vi "deleave.vi"(11 "Data":u64[](array[numeric])) -> (2 "Counts":i16[][](array[numeric]), 3 "Voltage":dbl[][](array[numeric]))   [LabVIEW 2015]
doc: "Deleave and convert Data. Deleaves data from DMA readout and converts with SubVIs to counts and voltages."
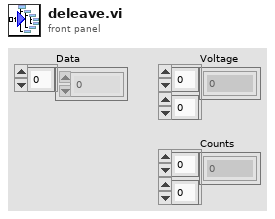
[diagram p1: front panel]
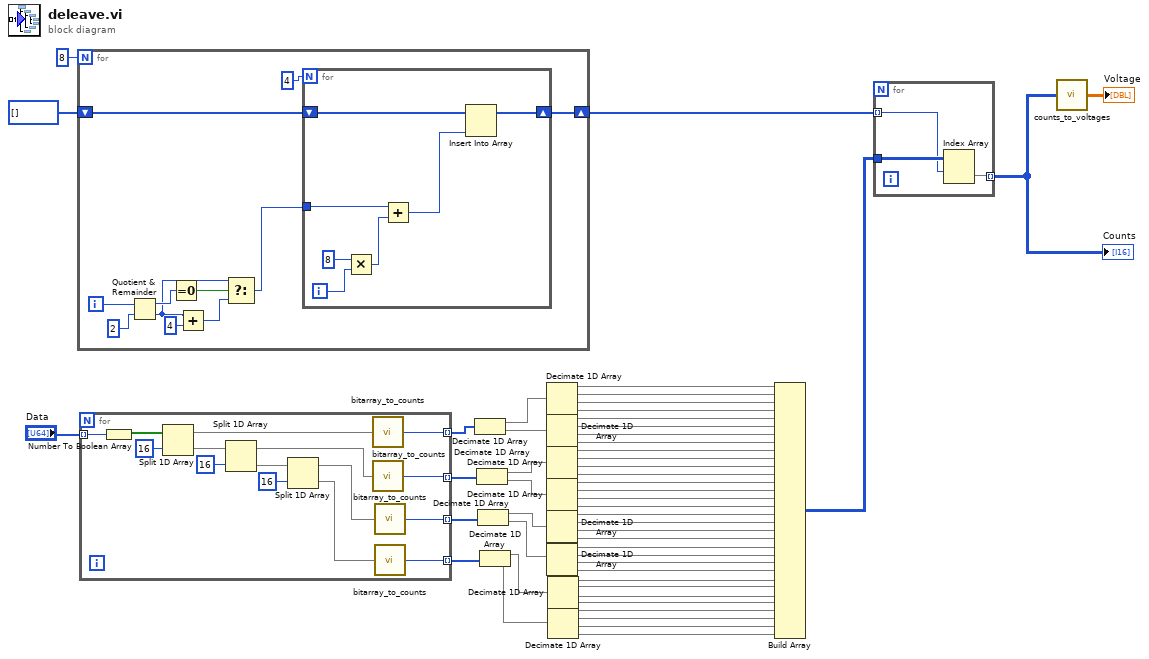
[diagram p0: block diagram]
diagram:
  n1 = for {
    N: 8 -> [_]
    shift-right: [w60] -> w2
    shift-left: i32[] [] -> [w61]
    i -> [w59]
    n2 = Quotient & Remainder(x=w59, y=2) -> (x-y*floor(x/y)=w57:i32, floor(x/y)=w52:i32)
    n3 = Equal To 0?(x=w57) -> (x = 0?=w55:bool)
    n4 = Add(x=w52, y=4) -> (x+y=w54:i32)
    n5 = Select(t=w52, s=w55, f=w54) -> (s? t:f=w53:i32)
    n6 = for {
      N: 4 -> [_]
      shift-right: [w64] -> w60
      shift-left: w61 -> [w65]
      tunnel: w53 -> [w69]
      i -> [w68]
      n7 = Multiply(x=8, y=w68) -> (x*y=w66:i32)
      n8 = Add(x=w69, y=w66) -> (x+y=w63:i32)
      n9 = Insert Into Array(array=w65, new element=w63) -> (w64:i32[])  [unwired: 1 in]
    }
  }
  n10 = for {
    tunnel: "Data" -> [w84] mode=indexing
    tunnel: [w76] -> w7 mode=indexing
    tunnel: [w74] -> w8 mode=indexing
    tunnel: [w72] -> w9 mode=indexing
    tunnel: [w71] -> w10 mode=indexing
    n11 = Number To Boolean Array(number=w84) -> (Boolean array=w83:bool[])
    n12 = Split 1D Array(array=w83, index=16) -> (first subarray=w77:bool[], second subarray=w81:bool[])
    n13 = Split 1D Array(array=w81, index=16) -> (first subarray=w75:bool[], second subarray=w78:bool[])
    n14 = Split 1D Array(array=w78, index=16) -> (first subarray=w73:bool[], second subarray=w70:bool[])
    n15 = call "bitarray_to_counts.vi"("16Bit Array"=w77) -> ("Counts"=w76:i16)
    n16 = call "bitarray_to_counts.vi"("16Bit Array"=w75) -> ("Counts"=w74:i16)
    n17 = call "bitarray_to_counts.vi"("16Bit Array"=w73) -> ("Counts"=w72:i16)
    n18 = call "bitarray_to_counts.vi"("16Bit Array"=w70) -> ("Counts"=w71:i16)
  }
  n19 = Decimate 1D Array(w7) -> (w11:i16[], w12:i16[])
  n20 = Decimate 1D Array(w8) -> (w14:i16[], w13:i16[])
  n21 = Decimate 1D Array(w9) -> (w15:i16[], w16:i16[])
  n22 = Decimate 1D Array(w10) -> (w17:i16[], w18:i16[])
  n23 = Decimate 1D Array(w11) -> (w19:i16[], w20:i16[], w21:i16[], w22:i16[])
  n24 = Decimate 1D Array(w12) -> (w23:i16[], w24:i16[], w25:i16[], w26:i16[])
  n25 = Decimate 1D Array(w14) -> (w27:i16[], w28:i16[], w29:i16[], w30:i16[])
  n26 = Decimate 1D Array(w13) -> (w31:i16[], w32:i16[], w33:i16[], w34:i16[])
  n27 = Decimate 1D Array(w15) -> (w35:i16[], w36:i16[], w37:i16[], w38:i16[])
  n28 = Decimate 1D Array(w16) -> (w39:i16[], w40:i16[], w41:i16[], w42:i16[])
  n29 = Decimate 1D Array(w17) -> (w43:i16[], w44:i16[], w45:i16[], w46:i16[])
  n30 = Decimate 1D Array(w18) -> (w47:i16[], w48:i16[], w49:i16[], w50:i16[])
  n31 = Build Array(w19, w20, w21, w22, w23, w24, w25, w26, w27, w28, w29, w30, w31, w32, w33, w34, w35, w36, w37, w38, w39, w40, w41, w42, w43, w44, w45, w46, w47, w48, w49, w50) -> (w3:i16[][])
  n32 = for {
    tunnel: w3 -> [w87]
    tunnel: w2 -> [w86] mode=indexing
    tunnel: [w85] -> w1 mode=indexing
    n33 = Index Array(array=w87, index (row)=w86) -> (element=w85:i16[])  [unwired: 1 in]
  }
  "Counts" <- w1
  n34 = call "counts_to_voltages.vi"("Count Array"=w1) -> ("Voltage Array"=→"Voltage":dbl[][])
